vi "Untitled 2 (SubVI).vi"(10 "Numeric in":i32, 11 "Boolean in":bool) -> (3 "Numeric out":i32)   [LabVIEW 2021]
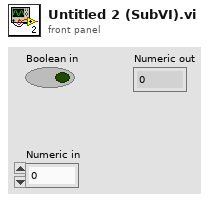
[diagram p1: front panel]
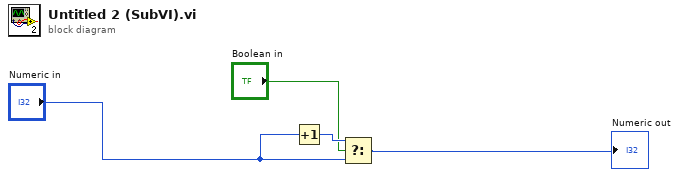
[diagram p0: block diagram]
diagram:
  n1 = Increment(x="Numeric in") -> (x+1=w3:i32)
  n2 = Select(t=w3, s="Boolean in", f="Numeric in") -> (s? t:f=→"Numeric out":i32)
